vi "SSC DAQmx Configure Regeneration.vi"(0 "DAQmx SSC in":T1[](array[typedef]), 5 "RegenMode":i32(ring)=10097 items=["Allow Regeneration"=10097, "Do Not Allow Regeneration"=10158], 11 "error in":errorcluster) -> (4 "DAQmx SSC out":T1[](array[typedef]), 15 "error out":errorcluster)   [LabVIEW 2020]
doc: "Specifies whether to allow NI-DAQmx to generate the same data multiple times."
uses:
  Pin Map/SSC DAQmx.ctl
  <resource>/objmgr/daqmx.rc
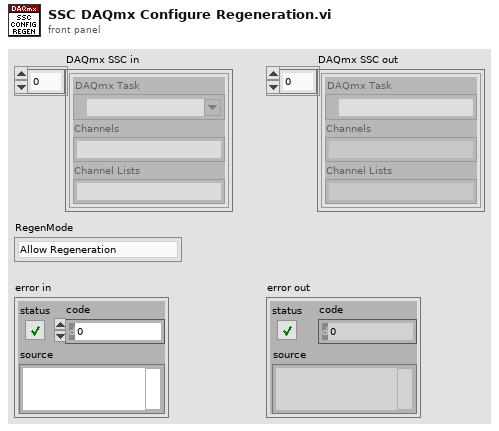
[diagram p1: front panel]
types:
  T1 = typedef "SSC DAQmx.ctl" = cluster{"DAQmx Task ":refnum<k21>, "Channels":string, "Channel Lists":string}
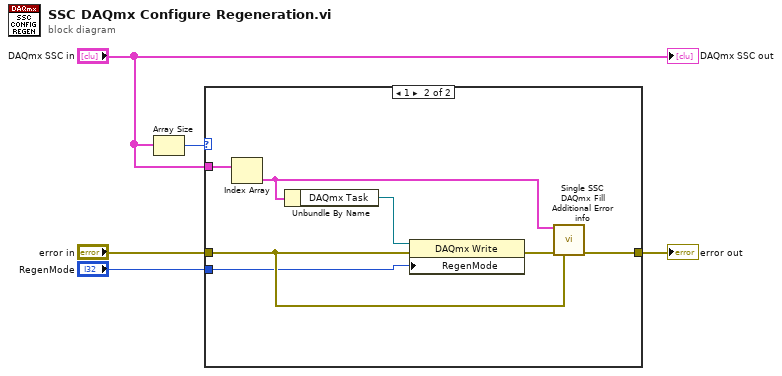
[diagram p0: block diagram]
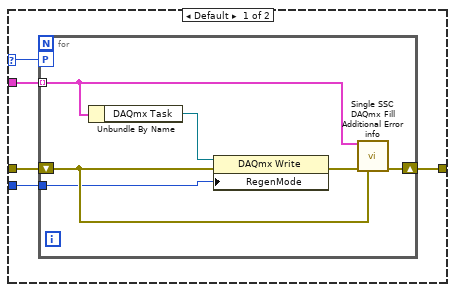
[diagram p2: hidden frame]
diagram:
  n1 = Array Size(array="DAQmx SSC in") -> (size(s)=w3:i32)
  n2 = case shown="1" w3 {
    selector: w3 -> [w8 _]
    tunnel: [w10 w23] -> w5
    tunnel: "error in" -> [w9 w22]
    tunnel: "DAQmx SSC in" -> [w7 w21]
    tunnel: "RegenMode" -> [w6 w20]
    frame Default {
      n3 = for {
        tunnel: w7 -> [w15] mode=indexing
        workers-P: w8 -> [_]
        shift-right: [w16] -> w10
        shift-left: w9 -> [w13]
        tunnel: w6 -> [w11]
        n4 = Unbundle By Name(w15) -> ("DAQmx Task"=w12:refnum<k21>)
        n5 = property class="DAQmx Write"(reference=w12, error in=w13, "RegenMode"=w11) -> (error out=w14:errorcluster)  [unwired: 1 out]
        n6 = call "Single SSC DAQmx Fill Additional Error info.vi"("DAQmx SSC in"=w15, "error in"=w14, "previous error in"=w13) -> ("error out"=w16:errorcluster)  [unwired: 12 in]
      }
    }
    frame 1 {
      n7 = Index Array(array=w21) -> (element=w17:T1)  [unwired: 1 in]
      n8 = Unbundle By Name(w17) -> ("DAQmx Task"=w18:refnum<k21>)
      n9 = property class="DAQmx Write"(reference=w18, error in=w22, "RegenMode"=w20) -> (error out=w19:errorcluster)  [unwired: 1 out]
      n10 = call "Single SSC DAQmx Fill Additional Error info.vi"("DAQmx SSC in"=w17, "error in"=w19, "previous error in"=w22) -> ("error out"=w23:errorcluster)  [unwired: 12 in]
    }
  }
  "error out" <- w5
  "DAQmx SSC out" <- "DAQmx SSC in"
